vi "Double_Card_Read_Ai.vi"(0 "dev":i32, 1 "每通道采样周期(s)":dbl, 2 "Points":u32, 3 "波形初始时间输入":timestamp, 5 "错误输入":errorcluster caption="错误输入（无错误）") -> (4 "波形初始时间输出":timestamp, 6 "Dev out":i32, 7 "数据输出":waveform(sgl)[](array[waveform]), 8 "error out":errorcluster caption="错误输出")   [LabVIEW 2018]
uses:
  WDT Get Final Time Value DBL.vi
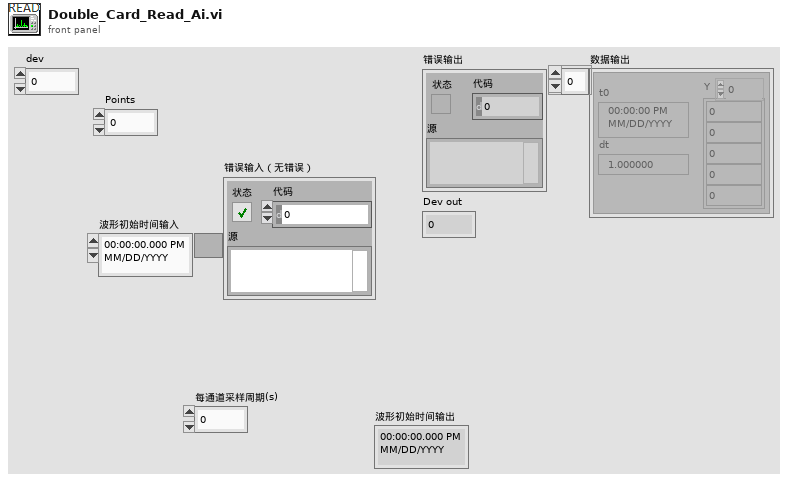
[diagram p1: front panel]
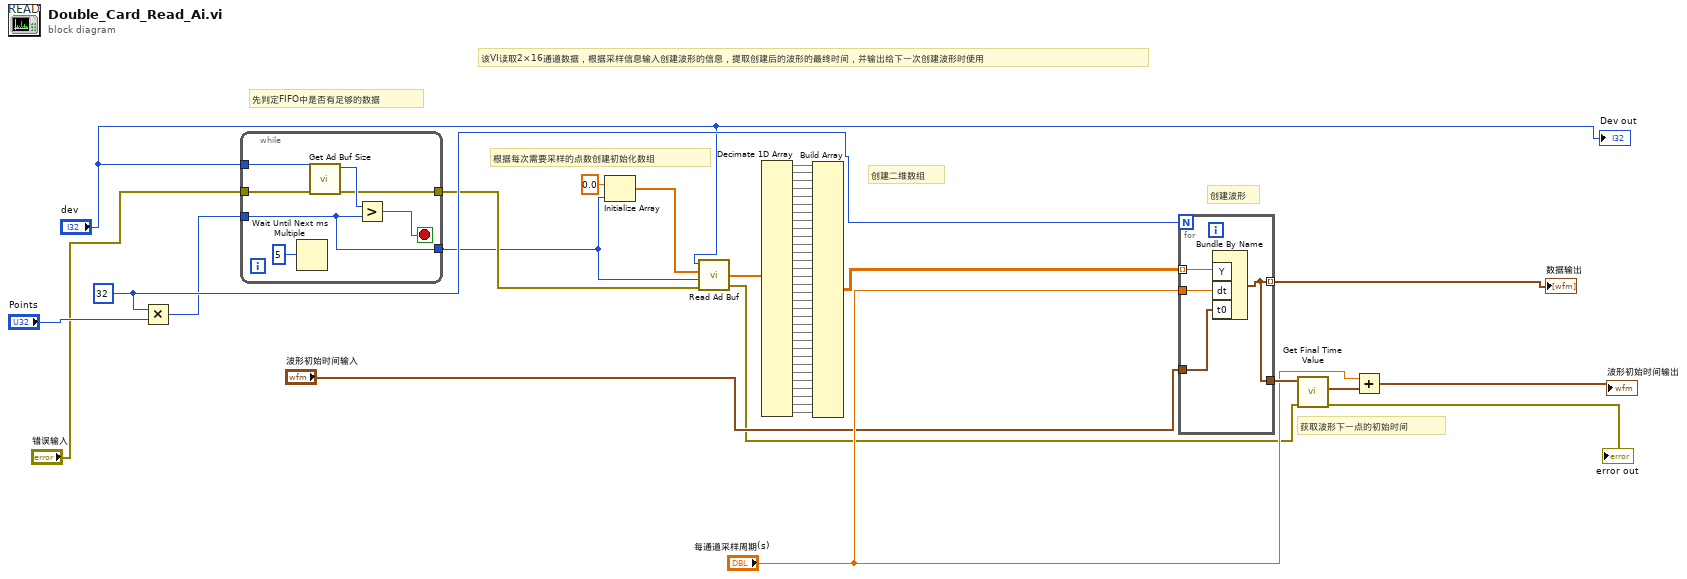
[diagram p0: block diagram]
diagram:
  w6 = u32 32 ("维数大小")
  # "先判定FIFO中是否有足够的数据"
  # "创建二维数组"
  # "该VI读取2×16通道数据，根据采样信息输入创建波形的信息，提取创建后的波形的最终时间，并输出给下一次创建波形时使用"
  # "获取波形下一点的初始时间"
  # "创建波形"
  # "根据每次需要采样的点数创建初始化数组"
  n1 = Multiply(x=w6, y="Points") -> (x*y=w4:u32)
  n2 = while {
    tunnel: "dev" -> [w53]
    tunnel: "错误输入" -> [w57]
    tunnel: w4 -> [w54]
    tunnel: [w56] -> w3
    tunnel: [w54] -> w2
    stop <- w55 stop-if-true
    n3 = Wait Until Next ms Multiple(millisecond multiple=u32 5) -> ()  [unwired: 1 out]
    n4 = call "Get Ad Buf Size.vi"("error in (no error)"=w57, "dev"=w53) -> ("error out"=w56:errorcluster, "function return"=w58:i32)  [unwired: 8 in]
    n5 = Greater?(x=w58, y=w54) -> (0:w55:bool)
  }
  n6 = Initialize Array(sgl 0.0 ("元素"), w2) -> (w45:sgl[])
  n7 = call "Read Ad Buf.vi"("error in (no error)"=w3, "num"=w2, "databuf"=w45, "dev"="dev") -> ("error out"=w8:errorcluster, "databuf out"=w43:sgl[])  [unwired: 1 out]
  n8 = Decimate 1D Array(w43) -> (w42:sgl[], w41:sgl[], w40:sgl[], w39:sgl[], w38:sgl[], w37:sgl[], w36:sgl[], w35:sgl[], w34:sgl[], w33:sgl[], w32:sgl[], w31:sgl[], w30:sgl[], w29:sgl[], w28:sgl[], w27:sgl[], w26:sgl[], w25:sgl[], w24:sgl[], w23:sgl[], w22:sgl[], w21:sgl[], w20:sgl[], w19:sgl[], w18:sgl[], w17:sgl[], w16:sgl[], w15:sgl[], w14:sgl[], w13:sgl[], w12:sgl[], w11:sgl[])
  n9 = Build Array(w42, w41, w40, w39, w38, w37, w36, w35, w34, w33, w32, w31, w30, w29, w28, w27, w26, w25, w24, w23, w22, w21, w20, w19, w18, w17, w16, w15, w14, w13, w12, w11) -> (w10:sgl[][])
  n10 = for {
    N: w6 -> [_]
    tunnel: w10 -> [w62] mode=indexing
    tunnel: [w61] -> w7 mode=indexing
    tunnel: [w61] -> w47
    tunnel: "每通道采样周期(s)" -> [w60]
    tunnel: "波形初始时间输入" -> [w59]
    n11 = Bundle By Name("Y"=w62, "dt"=w60, "t0"=w59) -> (w61:waveform(sgl))  [unwired: 1 in]
  }
  "数据输出" <- w7
  n12 = call-poly "Get Final Time Value.vi"("error in (no error)"=w8, "waveform in"=w47) -> ("error out"=→"error out":errorcluster, "tf"=w50:timestamp)  [unwired: 7 in, 1 out]
  n13 = Add(x="每通道采样周期(s)", y=w50) -> (x+y=→"波形初始时间输出":timestamp)
  "Dev out" <- "dev"
